vi "ReadRowRgbaU32.vi"(8 "error in":errorcluster, 10 "Row":i32, 11 "Image Reference In":T2) -> (0 "error out":errorcluster, 2 "Pixel Row":T1[](array[typedef]), 3 "Image Reference Out":T2)   [LabVIEW 2020, in "OpenLvVision_Image.lvlib" / "DataAccess.lvlib"]
doc: "Returns the values of an pixel row"
uses:
  DataAccess.lvlib
  Management/TypeDef/Image.ctl
  TypeDef/RgbaU32.ctl
  <vilib>/Utility/error.llb/Error Cluster From Error Code.vi
  <vilib>/ErrorRing/Error Ring.xnode
  Management/Management.lvlib
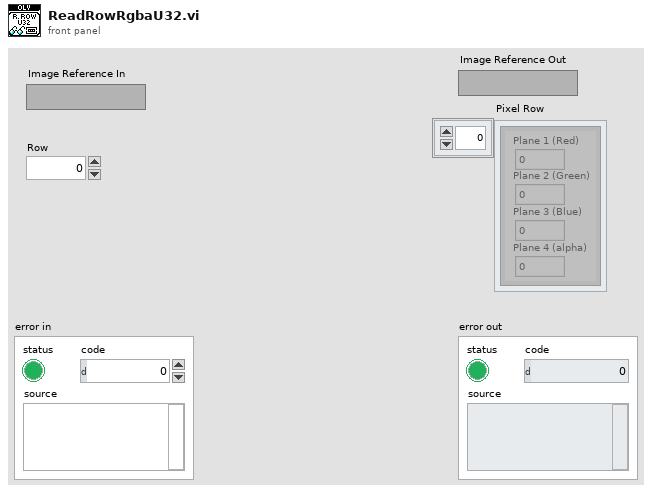
[diagram p1: front panel]
types:
  T1 = typedef "OpenLvVision_Image.lvlib/DataAccess.lvlib/RgbaU32.ctl" = cluster{"Plane 1 (Red)":u8, "Plane 2 (Green)":u8, "Plane 3 (Blue)":u8, "Plane 4 (alpha)":u8}
  T2 = typedef "OpenLvVision_Image.lvlib/Management.lvlib/Image.ctl" = refnum<image>
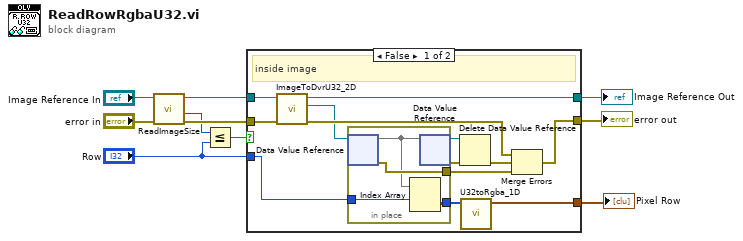
[diagram p0: block diagram]
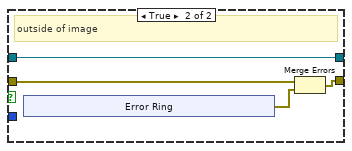
[diagram p2: hidden frame]
diagram:
  n1 = call "ReadImageSize.vi"("error in"="error in", "Image Reference In"="Image Reference In") -> ("error out"=w9:errorcluster, "Height"=w1:i32, "Image Reference Out"=w10:T2)  [unwired: 6 in, 1 out]
  n2 = Less Or Equal?(x=w1, y="Row") -> (x <= y?=w4:bool)
  n3 = case shown="False" w4 {
    tunnel: w10 -> [w23 w29]
    tunnel: w9 -> [w22 w31]
    tunnel: [w21 w29] -> w6
    tunnel: [w14 w28] -> w5
    tunnel: [w11 _] -> w2
    tunnel: "Row" -> [w13 _]
    frame False {
      # "inside image"
      n4 = call "ImageToDvrU32_2D.vi"("error in"=w22, "Image Reference In"=w23) -> ("error out"=w16:errorcluster, "EDVR 2D U32"=w15:refnum<data-value>, "Image Reference Out"=w21:T2)  [unwired: 6 in, 1 out]
      n5 = in-place {
        in-place-border: [w27] -> w19
        in-place-border: [w25] -> w12
        in-place-border: w13 -> [w24]
        n6 = in-place-dvr #1(w15) -> (w26:u32[][], w27:errorcluster)
        n7 = Index Array(array=w26, index (row)=w24) -> (element=w25:u32[])  [unwired: 1 in]
        n8 = in-place-dvr #1(w26) -> (w17:refnum<data-value>, w18:errorcluster)
      }
      n9 = Delete Data Value Reference(data value reference=w17, error in=w18) -> (error out=w20:errorcluster)  [unwired: 1 out]
      n10 = call "U32toRgba_1D.vi"("U32"=w12) -> ("Rgba"=w11:T1[])  [unwired: 10 in]
      n11 = Merge Errors(w16, w20, w19) -> (w14:errorcluster)
    }
    frame True {
      # "outside of image"
      n12 = xnode "Error Ring"() -> ("error out"=w30:errorcluster)
      n13 = Merge Errors(w31, w30) -> (w28:errorcluster)
    }
  }
  "error out" <- w5
  "Image Reference Out" <- w6
  "Pixel Row" <- w2
